vi "弹窗-配置过程错误.vi"(8 "error int":errorcluster caption="error in", 11 "当前配置流程":T1(ring)) -> ()   [LabVIEW 2013]
uses:
  <vilib>/sound2/lvsound2.llb/Sound File Info (path).vi
  <vilib>/sound2/lvsound2.llb/Sound File Read Open.vi
  <vilib>/sound2/lvsound2.llb/Sound File Read (DBL).vi
panel:
  out "标题":string
  out "提示语":string
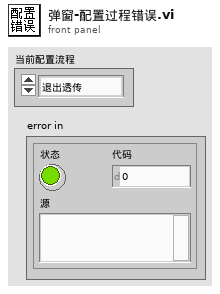
[diagram p1: front panel]
types:
  T1 = enum16{"退出透传", "进入AT指令", "退出AP连接", "设为STA", "连接指定AP", "设为STA开机自连", "获取MAC地址", "禁用智能连接", "透传接收", "连接至配置服务器", "进入透传发送", "等待云服务器端确认", "配置完成"}
  T2 = enum32{"Invalid", "Standard", "Closed", "Hidden", "Minimized", "Maximized"}
  T3 = typedef "Sound File Refnum.ctl" = refnum<file>
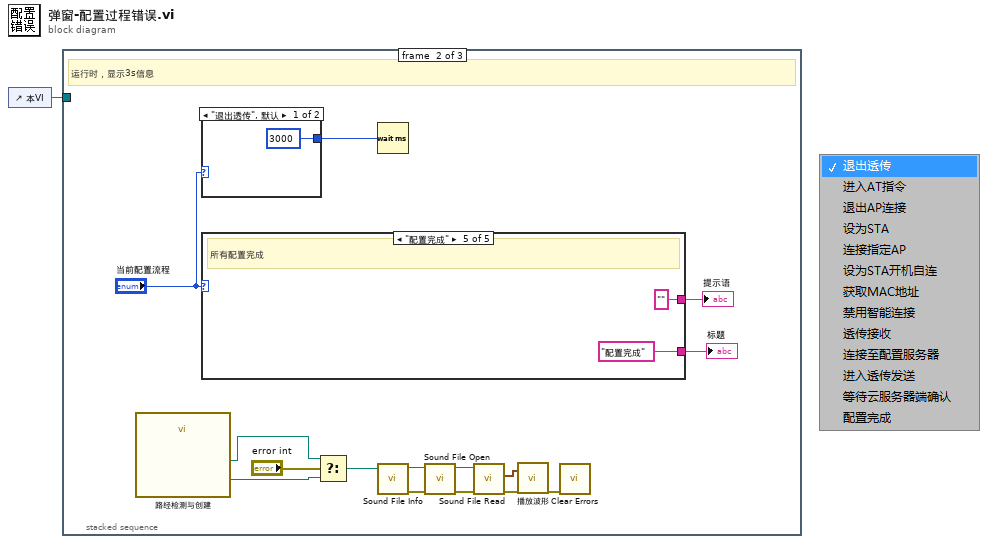
[diagram p0: block diagram]
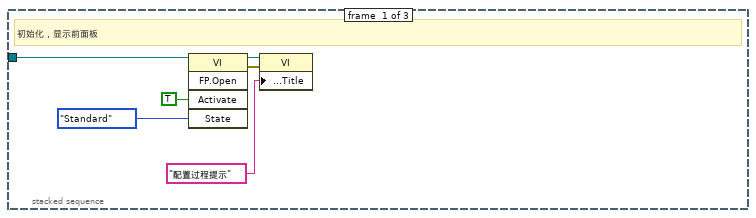
[diagram p2: hidden frame]
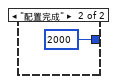
[diagram p3: hidden frame]
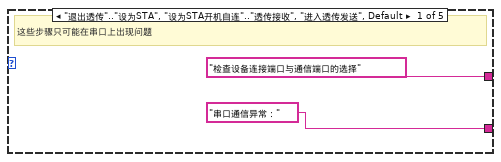
[diagram p4: hidden frame]
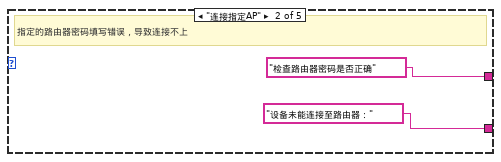
[diagram p5: hidden frame]
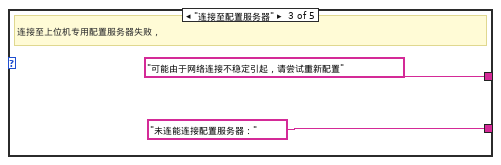
[diagram p6: hidden frame]
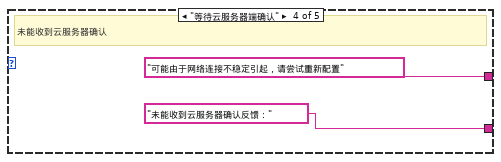
[diagram p7: hidden frame]
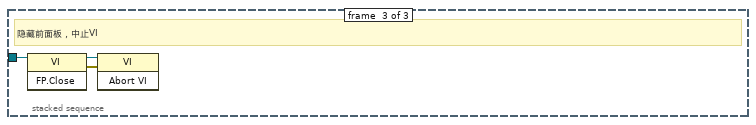
[diagram p8: hidden frame]
diagram:
  n1 = control-ref of="本VI"() -> (w1:refnum<vi>)
  n2 = stacked-sequence {
    tunnel: w1 -> [w7 _ w37]
    frame #0 {
      # "初始化，显示前面板"
      n3 = invoke class="VI" method="FP.Open"(reference=w7, "Activate"=TRUE ("激活？"), "State"=T2."Standard" ("状态")) -> (reference out=w4:refnum<vi>, error out=w3:errorcluster)  [unwired: 2 in, 3 out]
      n4 = property class="VI"(reference=w4, error in=w3, "Front Panel.Title"="配置过程提示" ("前面板窗口:标题")) -> ()  [unwired: 2 out]
    }
    frame #1 {
      # "运行时，显示3s信息"
      n5 = call "路经检测与创建.vi"() -> ("错误音效文件"=w17:path, "完成音效文件"=w16:path)  [unwired: 9 in, 1 out]
      n6 = case shown="\"退出透传\", 默认" "当前配置流程" {
        tunnel: [u32 3000 ("等待时间（毫秒）") u32 2000 ("等待时间（毫秒）")] -> w9
        frame "退出透传", Default {
        }
        frame "配置完成" {
        }
      }
      n7 = case shown="\"配置完成\"" "当前配置流程" {
        tunnel: ["检查设备连接端口与通信端口的选择" ("提示语") "检查路由器密码是否正确" ("提示语") "可能由于网络连接不稳定引起，请尝试重新配置" ("提示语") "可能由于网络连接不稳定引起，请尝试重新配置" ("提示语") "" ("提示语")] -> w11
        tunnel: ["串口通信异常：" ("提示语") "设备未能连接至路由器：" ("提示语") "未连能连接配置服务器：" ("提示语") "未能收到云服务器确认反馈：" ("提示语") "配置完成" ("提示语")] -> w8
        frame "退出透传".."设为STA", "设为STA开机自连".."透传接收", "进入透传发送", Default {
          # "这些步骤只可能在串口上出现问题"
        }
        frame "连接指定AP" {
          # "指定的路由器密码填写错误，导致连接不上"
        }
        frame "连接至配置服务器" {
          # "连接至上位机专用配置服务器失败，"
        }
        frame "等待云服务器端确认" {
          # "未能收到云服务器确认"
        }
        frame "配置完成" {
          # "所有配置完成"
        }
      }
      "提示语" <- w11
      "标题" <- w8
      n8 = Select(t=w17, s="error int", f=w16) -> (s? t:f=w15:path)
      n9 = Wait (ms)(milliseconds to wait=w9) -> ()  [unwired: 1 out]
      n10 = call-poly <vilib>:"Sound File Info.vi"("path"=w15) -> ("error out"=w20:errorcluster, "path out"=w21:path)  [unwired: 7 in, 2 out]
      n11 = call-poly <vilib>:"Sound File Open.vi"("error in (no error)"=w20, "path"=w21) -> ("error out"=w19:errorcluster, "sound file refnum"=w22:T3)  [unwired: 8 in]
      n12 = call-poly <vilib>:"Sound File Read.vi"("error in (no error)"=w19, "sound file refnum"=w22) -> ("error out"=w13:errorcluster, "data"=w14:waveform(dbl)[])  [unwired: 5 in, 3 out]
      n13 = call "播放波形"("Data"=w14, "error in"=w13) -> ("error out"=w12:errorcluster)  [unwired: 17 in]
      n14 = call <vilib>:"Clear Errors.vi"("error in (no error)"=w12) -> ()  [unwired: 6 in, 1 out]
    }
    frame #2 {
      # "隐藏前面板，中止VI"
      n15 = invoke class="VI" method="FP.Close"(reference=w37) -> (reference out=w36:refnum<vi>, error out=w35:errorcluster)  [unwired: 2 in, 1 out]
      n16 = invoke class="VI" method="Abort VI"(reference=w36, error in=w35) -> ()  [unwired: 1 in, 3 out]
    }
  }
